vi "WriteData.vi"(8 "error in (no error)":errorcluster, 10 "Data":T1, 11 "DataBank in":refnum<class "DataBank.lvclass">) -> (0 "error out":errorcluster, 3 "DataBank out":refnum<class "DataBank.lvclass">)   [LabVIEW 2012, in "DataBank.lvclass"]
uses:
  DataBank.lvclass
  DataBank.lvclass/DataBank.ctl
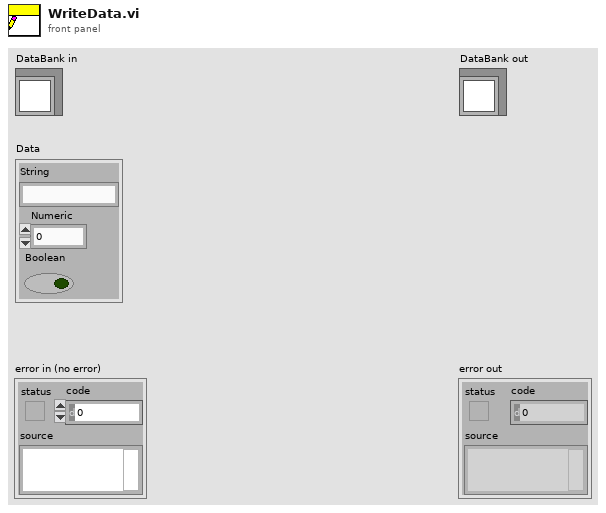
[diagram p1: front panel]
types:
  T1 = cluster{"String":string, "Numeric":i32, "Boolean":bool}
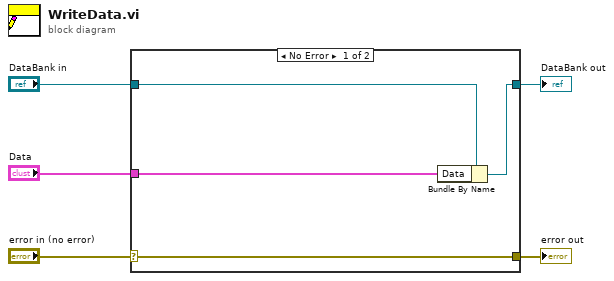
[diagram p0: block diagram]
diagram:
  n1 = case shown="No Error" "error in (no error)" {
    selector: "error in (no error)" -> [w9 w10]
    tunnel: [w9 w10] -> w4
    tunnel: [w7 w11] -> w2
    tunnel: "DataBank in" -> [w8 w11]
    tunnel: "Data" -> [w6 _]
    frame No Error {
      n2 = Bundle By Name(cluster=w8, "Data"=w6) -> (w7:refnum<class "DataBank.lvclass">)
    }
    frame Error {
    }
  }
  "error out" <- w4
  "DataBank out" <- w2
